vi "PumpOFF.vi"(8 "Error In":errorcluster, 10 "delay before read (ms)":u32=500, 11 "VISA resource name":refnum<visa-resource-name>="COM7") -> (0 "Error Out":errorcluster, 1 "Write byte count":u32, 2 "Read byte count":u32, 3 "read buffer":string)   [LabVIEW 2016]
uses:
  <vilib>/Instr/_visa.llb/VISA Configure Serial Port (Instr).vi
panel:
  out "Bytes read":u32
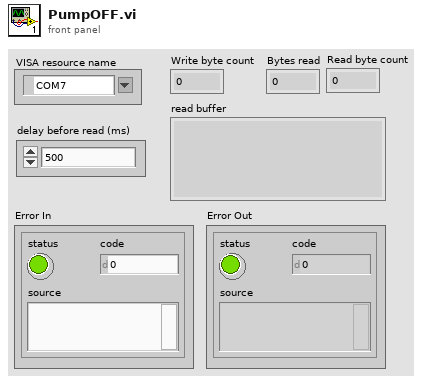
[diagram p1: front panel]
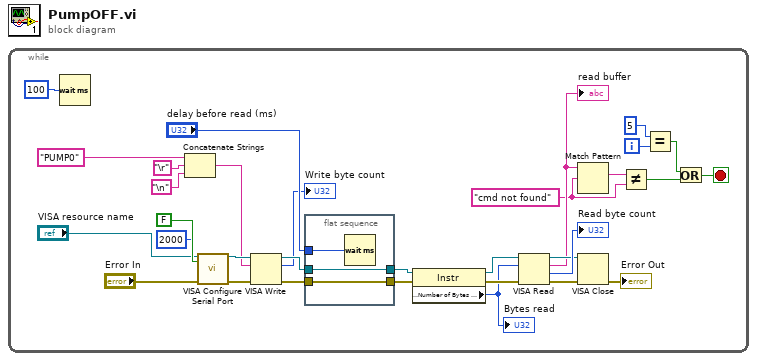
[diagram p0: block diagram]
diagram:
  n1 = while {
    i -> [w5]
    stop <- w1 stop-if-true
    w6 = "cmd not found" ("regular expression")
    n2 = Wait (ms)(milliseconds to wait=u32 100) -> ()  [unwired: 1 out]
    n3 = Concatenate Strings("PUMP0" ("Command"), "\r", "\n") -> (w25:string)
    n4 = call-poly "VISA Configure Serial Port"("VISA resource name"="VISA resource name", "timeout (10sec)"=u32 2000, "Enable Termination\nChar (T)"=FALSE ("Enable Termination\nChar (T)"), "error in (no error)"="Error In") -> ("VISA resource name out"=w26:refnum<visa-resource-name>, "error out"=w24:errorcluster)  [unwired: 5 in, 5 out]
    n5 = VISA Write(VISA resource name=w26, write buffer=w25, error in (no error)=w24) -> (VISA resource name out=w22:refnum<visa-resource-name>, return count=→"Write byte count":u32, error out=w21:errorcluster)
    n6 = flat-sequence {
      tunnel: w21 -> [w34]
      tunnel: [w34] -> w19
      tunnel: w22 -> [w33]
      tunnel: [w33] -> w18
      tunnel: "delay before read (ms)" -> [w35]
      frame #0 {
        n7 = Wait (ms)(milliseconds to wait=w35) -> ()  [unwired: 1 out]
      }
    }
    n8 = property class="Instr"(reference=w18, error in=w19) -> (reference out=w14:refnum<visa-resource-name>, error out=w13:errorcluster, "Serial Settings:Number of Bytes at Serial Port"=w12:u32)
    "Bytes read" <- w12
    n9 = VISA Read(VISA resource name=w14, byte count=w12, error in (no error)=w13) -> (VISA resource name out=w16:refnum<visa-resource-name>, read buffer=w8:string, return count=→"Read byte count":u32, error out=w15:errorcluster)
    "read buffer" <- w8
    n10 = Match Pattern(string=w8, regular expression=w6) -> (match substring=w7:string)  [unwired: 1 in, 3 out]
    n11 = VISA Close(VISA resource name=w16, error in (no error)=w15) -> (error out=→"Error Out":errorcluster)
    n12 = Not Equal?(x=w7, y=w6) -> (x != y?=w2:bool)
    n13 = Equal?(x=5, y=w5) -> (x = y?=w3:bool)
    n14 = Or(x=w3, y=w2) -> (x .or. y?=w1:bool)
  }
